vi "Clear Report Text.vi"(0 "report in":refnum<class "NI_HTML.lvclass">, 11 "error in (no error)":errorcluster) -> (4 "report out":refnum<class "NI_HTML.lvclass">, 15 "error out":errorcluster)   [LabVIEW 2020, in "NI_HTML.lvclass"]
doc: "Clears the text and related formatting information from the report. You cannot use this VI with Word and Excel reports."
uses:
  NI_HTML.lvclass
  NI_HTML.lvclass/NI_HTML.ctl
  NI_ReportGenerationCore.lvlib
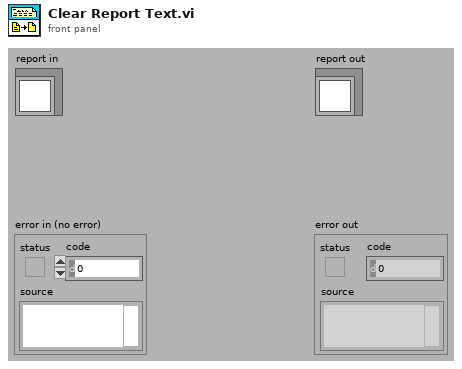
[diagram p1: front panel]
types:
  T1 = typedef "NI_ReportGenerationCore.lvlib/HTML Report Data.ctl" = cluster{"Body Text":string, "Font Tag":string, "Title Text":string, "Header Text":string, "Footer Text":string, "Image List":path[]}
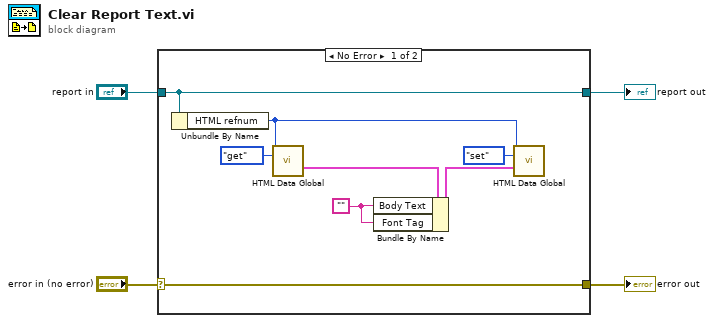
[diagram p0: block diagram]
diagram:
  n1 = case shown="No Error" "error in (no error)" {
    selector: "error in (no error)" -> [w11 w14]
    tunnel: [w11 w14] -> w3
    tunnel: [w8 w13] -> w1
    tunnel: "report in" -> [w8 w13]
    frame No Error {
      w12 = ""
      n2 = Unbundle By Name(w8) -> ("HTML refnum"=w5:u32)
      n3 = call "HTML Data Global.vi"("HTML refnum"=w5, "menu"=enum16{"init", "get", "set", "delete"}."get") -> ("HTML report data out"=w7:T1)  [unwired: 1 in, 12 out]
      n4 = Bundle By Name(cluster=w7, "Body Text"=w12, "Font Tag"=w12) -> (w6:T1)
      n5 = call "HTML Data Global.vi"("HTML refnum"=w5, "menu"=enum16{"init", "get", "set", "delete"}."set", "HTML report data in"=w6) -> ()  [unwired: 13 out]
    }
    frame Error {
    }
  }
  "error out" <- w3
  "report out" <- w1
